vi "Release-filter-file.vi"(8 "error in":errorcluster, 11 "Data ref. in":refnum<data-value>) -> (0 "error IO":errorcluster, 1 "Succes?":bool, 3 "Data ref.":refnum<data-value>)   [LabVIEW 2013, in "CameraVision.lvlib" / "CV-Main.lvclass"]
doc: "This function closes the access references to the characteristics data file. This prevents further changes and allows the memory to be released.\n\nIn case the acquisition was aborted in the initialization phase, the references could be invalid. Invalid references are detected and ignored."
uses:
  CV-Main.lvclass
  UI/Module-states.ctl
  CV-Main.lvclass/CV-Main.ctl
  Filter/CV-Filter.lvclass/CV-Filter.ctl
  Read Filter params.vi
  Filter/Read Filter file reference.vi
  Filter/CV-Filter.lvclass
  UI/CV-UI.lvclass
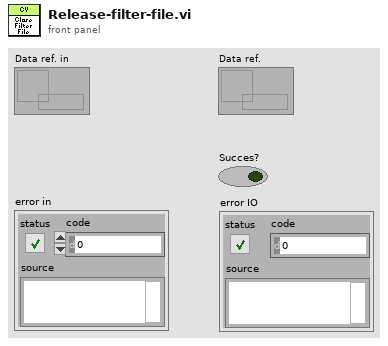
[diagram p1: front panel]
types:
  T1 = typedef "CameraVision.lvlib/CV-UI.lvclass/Module-states.ctl" = enum16{"Inactive", "Active", "Data-loss", "Error", "Simulation", "Synchronizing", "Initialized", "Released"}
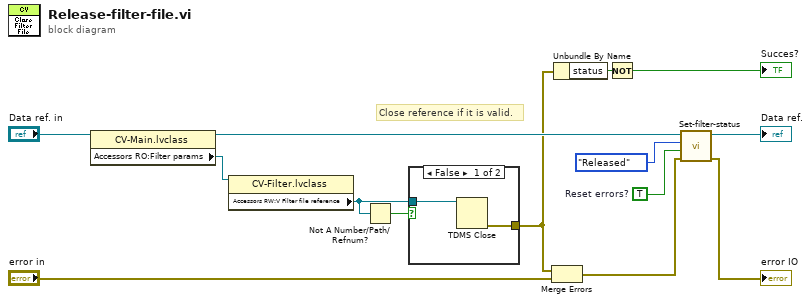
[diagram p0: block diagram]
diagram:
  w1 = TRUE  # Reset errors?
  # "Close reference if it is valid."
  n1 = property class="CV-Main.lvclass"(reference="Data ref. in") -> (reference out=w8:refnum<data-value>, "Accessors RO:Filter params"=w5:refnum<data-value>)  [unwired: 1 in, 1 out]
  n2 = property class="CV-Filter.lvclass"(reference=w5) -> ("Accessors RW:V Filter file reference"=w6:refnum<k34>)  [unwired: 1 in, 2 out]
  n3 = Not A Number/Path/Refnum?(number/path/refnum=w6) -> (NaN/Path/Refnum?=w7:bool)
  n4 = case shown="False" w7 {
    tunnel: [w16 _] -> w3
    tunnel: w6 -> [w15 _]
    frame False {
      n5 = TDMS Close(11:w15) -> (0:w16:errorcluster)  [unwired: 1 in, 1 out]
    }
    frame True {
    }
  }
  n6 = Merge Errors(w3, "error in") -> (w4:errorcluster)
  n7 = Unbundle By Name(w3) -> ("status"=w9:bool)
  n8 = Not(x=w9) -> (.not. x?=→"Succes?":bool)
  n9 = call "Set-filter-status.vi"("error in"=w4, "Reset errors?"=w1, "Filter status in"=Module-states."Released" ("Acquisition status"), "Data ref. in"=w8) -> ("error IO"=→"error IO":errorcluster, "Data ref."=→"Data ref.":refnum<data-value>)  [unwired: 5 in, 1 out]
